vi "updateDataPoints.vi"(8 "error in (no error)":errorcluster, 9 "Force Measured":dbl[unit] min=-888.0 max=888.0 format="%.2f", 10 "Distance Measured":dbl[unit]=1.0 min=1.0 max=300.0 format="%.1f", 11 "StiffnessCalculator in":refnum<class "StiffnessCalculator.lvclass">) -> (0 "error out":errorcluster, 2 "stiffnessCalculated":dbl[unit], 3 "StiffnessCalculator out":refnum<class "StiffnessCalculator.lvclass">)   [LabVIEW 2015, in "StiffnessCalculator.lvclass"]
uses:
  StiffnessCalculator.lvclass
  StiffnessCalculator.lvclass/StiffnessCalculator.ctl
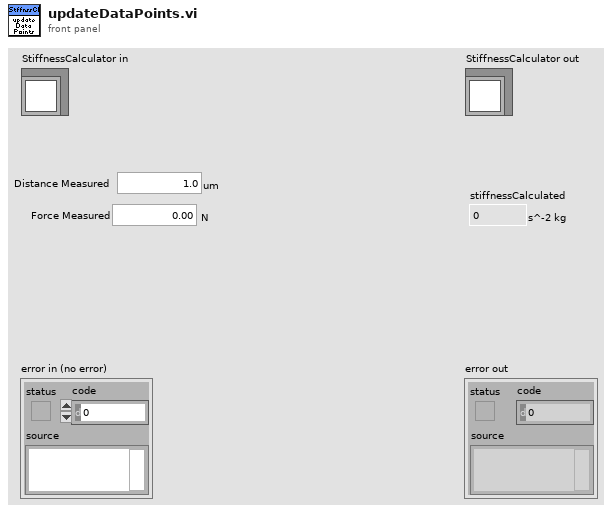
[diagram p1: front panel]
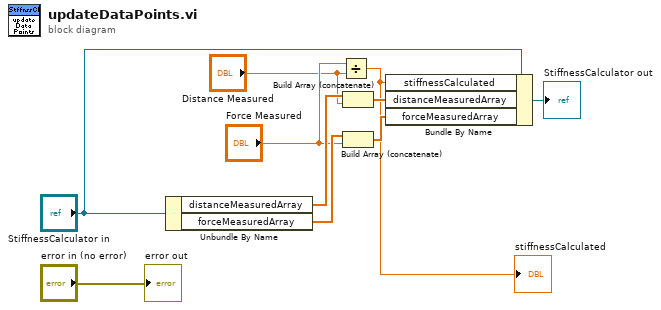
[diagram p0: block diagram]
diagram:
  n1 = Unbundle By Name("StiffnessCalculator in") -> ("distanceMeasuredArray"=w7:dbl[unit][], "forceMeasuredArray"=w5:dbl[unit][])
  n2 = Divide(x="Force Measured", y="Distance Measured") -> (x/y=w1:dbl[unit])
  "stiffnessCalculated" <- w1
  n3 = Build Array (concatenate)(w7, "Distance Measured") -> (w6:dbl[unit][])
  n4 = Build Array (concatenate)(w5, "Force Measured") -> (w4:dbl[unit][])
  n5 = Bundle By Name(cluster="StiffnessCalculator in", "stiffnessCalculated"=w1, "distanceMeasuredArray"=w6, "forceMeasuredArray"=w4) -> (→"StiffnessCalculator out":refnum<class "StiffnessCalculator.lvclass">)
  "error out" <- "error in (no error)"
